vi "ExtractControlRefRecursive.vi"(6 "HierarchyLevel":i32, 8 "error in (no error)":errorcluster, 10 "ParentName":string, 11 "Controls[]":refnum<vi>[](array[refnum])) -> (0 "error out":errorcluster, 3 "Array":T1[](array[typedef]))   [LabVIEW 2020, in "ContextHelpEditor.lvlib"]
uses:
  ContextHelpEditor.lvlib
  ControlRef--cluster.ctl
  <vilib>/picture/picture.llb/imagedata.ctl
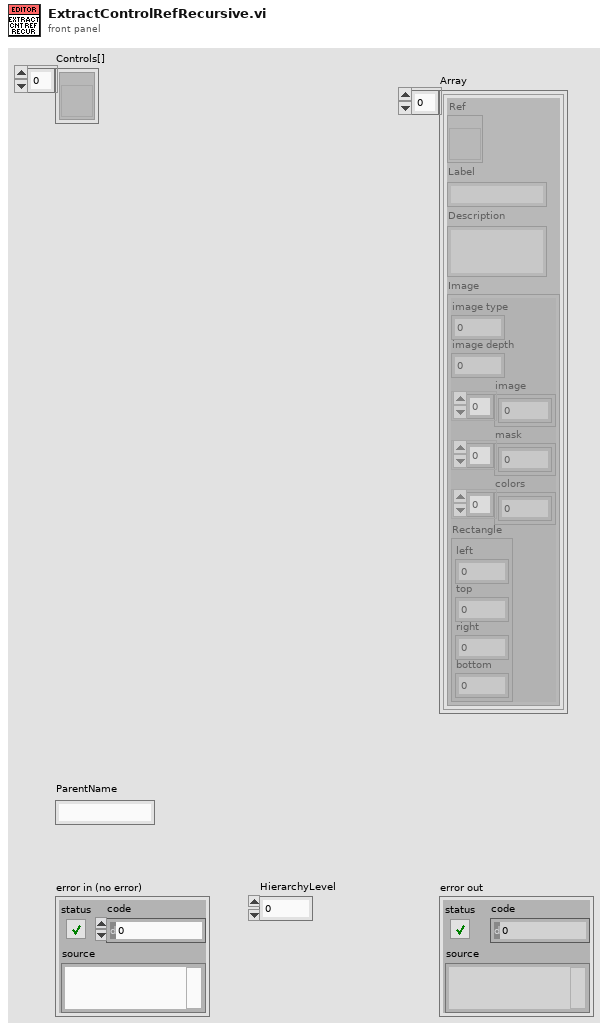
[diagram p1: front panel]
types:
  T1 = typedef "ContextHelpEditor.lvlib/ControlRef--cluster.ctl" = cluster{"Ref":refnum<vi>, "Label":string, "Description":string, "Image":T2}
  T2 = typedef "imagedata.ctl" = cluster{"image type":i32, "image depth":i32, "image":u8[], "mask":u8[], "colors":u32[], "Rectangle":cluster{"left":i16, "top":i16, "right":i16, "bottom":i16}}
  T3 = enum32{"not a typedef", "typedef", "strict typedef", "class private data"}
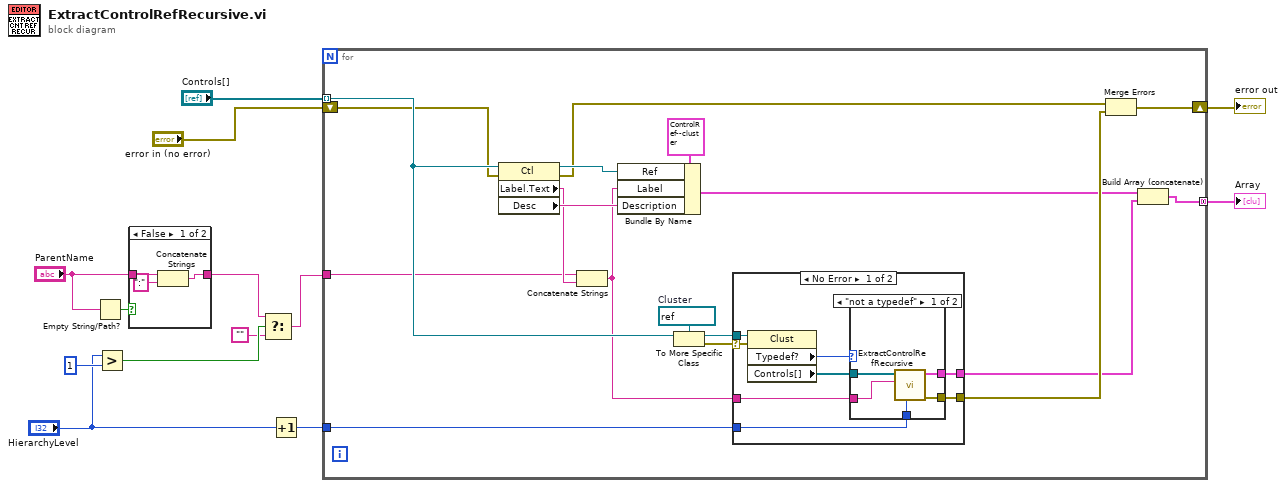
[diagram p0: block diagram]
diagram:
  n1 = Empty String/Path?(string/path="ParentName") -> (empty?=w5:bool)
  n2 = Greater?(x="HierarchyLevel", y=1) -> (0:w4:bool)
  n3 = case shown="False" w5 {
    tunnel: "ParentName" -> [w16 w17]
    tunnel: [w14 w17] -> w3
    frame False {
      n4 = Concatenate Strings(w16, ":" ("string")) -> (w14:string)
    }
    frame True {
    }
  }
  n5 = Select(t=w3, s=w4, f="") -> (s? t:f=w2:string)
  n6 = Increment(x="HierarchyLevel") -> (x+1=w6:i32)
  n7 = for {
    tunnel: "Controls[]" -> [w35] mode=indexing
    tunnel: [w34] -> w12 mode=concatenating
    shift-right: [w32] -> w13
    shift-left: "error in (no error)" -> [w33]
    tunnel: w2 -> [w20]
    tunnel: w6 -> [w18]
    w27 = refnum<vi> refnum  # Cluster
    n8 = property class="Ctl"(reference=w35, error in=w33) -> (reference out=w30:refnum<vi>, error out=w28:errorcluster, "Label.Text"=w21:string, "Desc"=w29:string)
    n9 = Concatenate Strings(w20, w21) -> (w19:string)
    n10 = Bundle By Name(cluster=T1 {"Ref"=refnum, "Label"="", "Description"="", "Image"={"image type"=0, "image depth"=0, "image"=[], "mask"=[], "colors"=[], "Rectangle"={"left"=0, "top"=0, "right"=0, "bottom"=0}}} ("ControlRef"), "Ref"=w30, "Label"=w19, "Description"=w29) -> (w23:T1)
    n11 = To More Specific Class(target class=w27, reference=w35) -> (specific class reference=w26:refnum<vi>, error out=w25:errorcluster)  [unwired: 1 in]
    n12 = case shown="No Error" w25 {
      selector: w25 -> [w42 _]
      tunnel: w26 -> [w43 _]
      tunnel: w19 -> [w39 _]
      tunnel: [w38 _] -> w22
      tunnel: [w37 _] -> w24
      tunnel: w18 -> [w36 _]
      frame No Error {
        n13 = property class="Clust"(reference=w43, error in=w42) -> ("Typedef?"=w41:T3, "Controls[]"=w40:refnum<vi>[])  [unwired: 2 out]
        n14 = case shown="\"not a typedef\"" w41 {
          tunnel: w40 -> [w48 _]
          tunnel: w39 -> [w47 _]
          tunnel: [w46 _] -> w38
          tunnel: [w45 _] -> w37
          tunnel: w36 -> [w44 _]
          frame "not a typedef" {
            n15 = call "ExtractControlRefRecursive.vi"("HierarchyLevel"=w44, "ParentName"=w47, "Controls[]"=w48) -> ("error out"=w45:errorcluster, "Array"=w46:T1[])  [unwired: 7 in]
          }
          frame Default {
          }
        }
      }
      frame Error {
      }
    }
    n16 = Merge Errors(w28, w24) -> (w32:errorcluster)
    n17 = Build Array (concatenate)(w23, w22) -> (w34:T1[])
  }
  "error out" <- w13
  "Array" <- w12
